vi "StopProgram.vi"(8 "error in (no error)":errorcluster, 9 "taskId":i32(ring) items=["TLibrary", "T01", "T02", "T03", "T04", "T05", "T06", "T07", "T08", "T09", "T10", "T11", "T12", "T13", "T14", "T15", "T16", "T17", "T18", "T19", "T20", "T21", "T22", "T23", "T24", "T25", "T26", "T27", "T28", "T29", "T30", "T31"], 11 "controller in":refnum<k24>) -> (0 "error out":errorcluster, 3 "controller out":refnum<k24>)   [LabVIEW 2016]
uses:
  C:/Users/TTUHEP/Documents/LabVIEW/2010/Bin/Aerotech.A3200.dll
  Bin/Aerotech.A3200.dll
  C:/Users/TTUHEP/Documents/LabVIEW/2010/Bin/Aerotech.A3200.LabVIEW.dll
  Bin/Aerotech.A3200.LabVIEW.dll
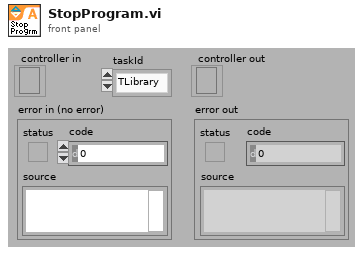
[diagram p1: front panel]
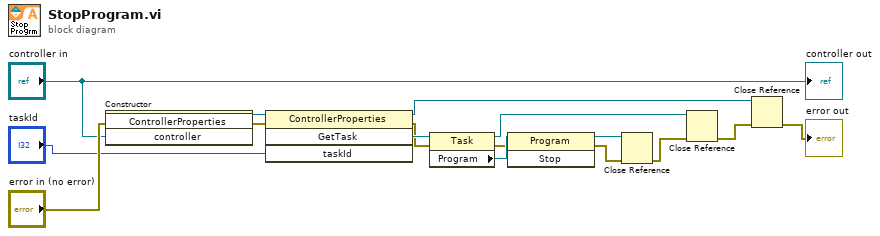
[diagram p0: block diagram]
diagram:
  n1 = constructor class="ControllerProperties"(error in="error in (no error)", "controller"="controller in") -> (reference out=w14:refnum<k24>, error out=w13:errorcluster)  [unwired: 2 in, 2 out]
  n2 = invoke class="ControllerProperties" method="GetTask"(reference=w14, error in=w13, "taskId"="taskId") -> (reference out=w12:refnum<k24>, error out=w6:errorcluster, "GetTask"=w7:refnum<k24>)  [unwired: 1 in, 1 out]
  n3 = property class="Task"(reference=w7, error in=w6) -> (reference out=w2:refnum<k24>, error out=w4:errorcluster, "Program"=w5:refnum<k24>)
  n4 = invoke class="Program" method="Stop"(reference=w5, error in=w4) -> (reference out=w8:refnum<k24>, error out=w9:errorcluster)  [unwired: 1 in, 1 out]
  n5 = Close Reference(reference=w8, error in (no error)=w9) -> (error out=w10:errorcluster)
  n6 = Close Reference(reference=w2, error in (no error)=w10) -> (error out=w3:errorcluster)
  n7 = Close Reference(reference=w12, error in (no error)=w3) -> (error out=→"error out":errorcluster)
  "controller out" <- "controller in"
